vi "itc_collect_auxPixelEvents.vi"   [LabVIEW 2016]
uses:
  <vilib>/rvi/DataTransferAndStorage/Container/XNode/niFpgaContainer.xnode
  <vilib>/eio/EIONode/EIONode.xnode
  <vilib>/rvi/eio/common/nirviEmuTemplateMethod_errors.vi
  <vilib>/rvi/FIFO/Fifo_Resource/nirvififoEmulationRead.vi
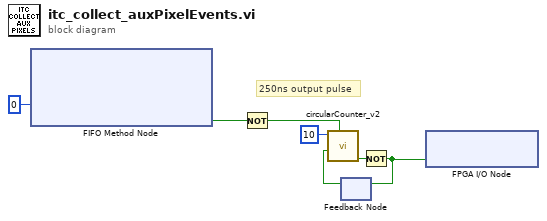
[diagram p0: block diagram]
diagram:
  # "250ns output pulse"
  n1 = xnode ("FIFO Method Node")("Timeout"=0) -> ("Timed Out?"=w1:bool)  [unwired: 1 in, 2 out]
  n2 = Not(x=w1) -> (.not. x?=w5:bool)
  n3 = feedback #1() -> (w3:bool)  [unwired: 1 in]
  n4 = call "circularCounter_v2.vi"("reset"=w5, "doStep"=w3, "maxCount"=u16 10) -> ("maxReached"=w4:bool)  [unwired: 5 in, 3 out]
  n5 = Not(x=w4) -> (.not. x?=w2:bool)
  n6 = feedback-in #1(w2) -> ()
  n7 = xnode "FPGA I/O Node"("pixelSyncAux"=w2) -> ()  [unwired: 1 in, 1 out]
